vi "ADAM_info_to_Raw_data_header.vi"(4 "Results file":path) -> ()   [LabVIEW 2010]
panel:
  out "ADAM Channel Info":string[][](table)
  out "Raw data filenames":string[](array[string])
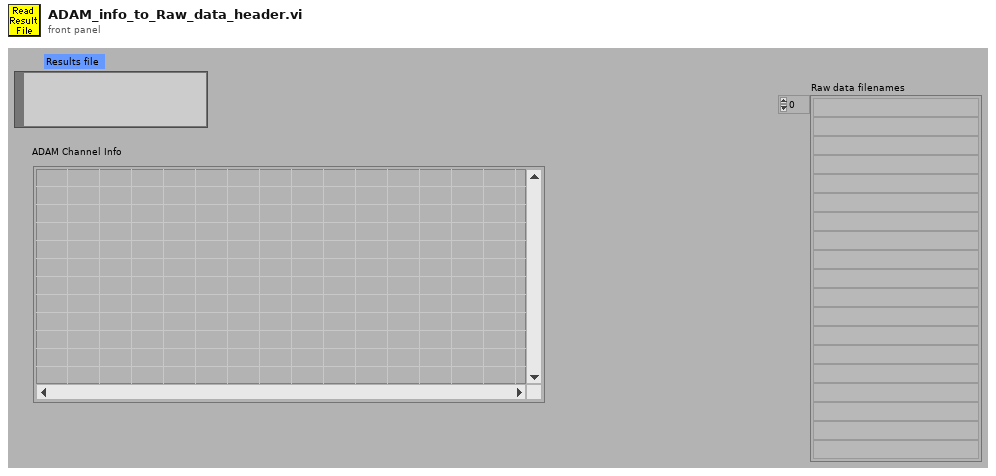
[diagram p1: front panel]
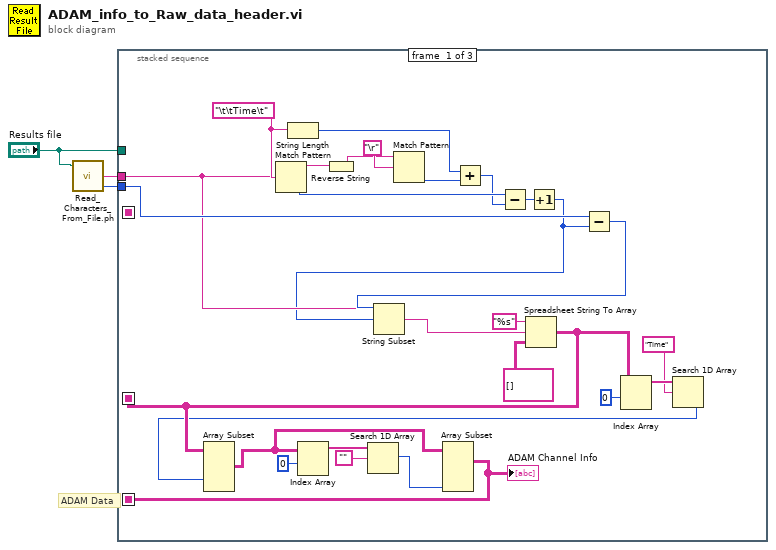
[diagram p0: block diagram]
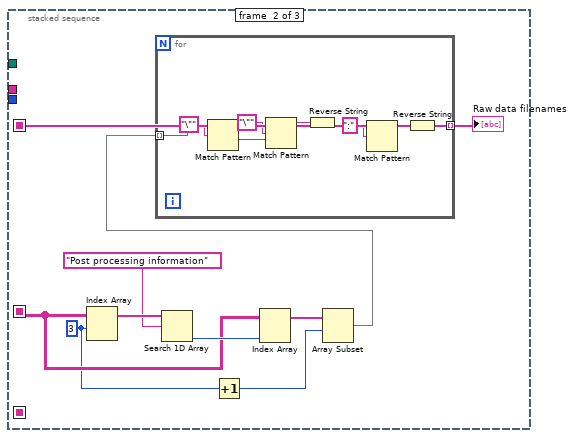
[diagram p2: hidden frame]
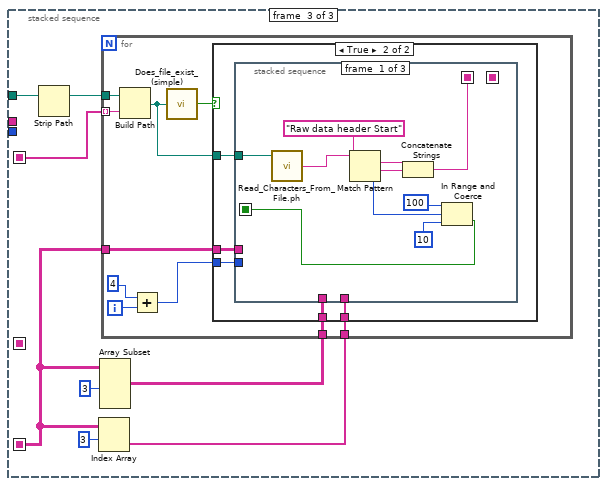
[diagram p3: hidden frame]
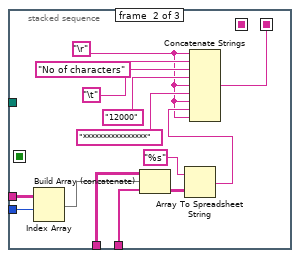
[diagram p5: hidden frame]
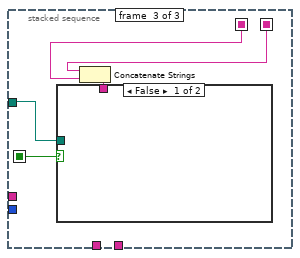
[diagram p6: hidden frame]
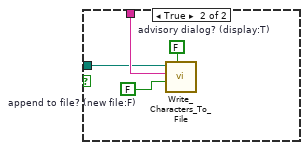
[diagram p7: hidden frame]
diagram:
  # "ADAM Data"
  n1 = call "Read_Characters_From_File.ph.vi"("file path (dialog if empty)"="Results file") -> ("character string"=w3:string, "mark after read (chars.)"=w2:i32)  [unwired: 5 in, 2 out]
  n2 = stacked-sequence {
    seq-local: [w7 _ _] -> [_ w36 _]
    seq-local: [w9 _ _] -> [_ _ w51]
    seq-local: [_ w31 _] -> [_ _ w53]
    tunnel: w3 -> [w19 _ _]
    tunnel: w2 -> [w22 _ _]
    tunnel: "Results file" -> [_ _ w54]
    frame #0 {
      w27 = "\t\tTime\t" ("regular expression")
      n3 = Match Pattern(string=w19, regular expression=w27) -> (before substring=w30:string, offset past match=w24:i32)  [unwired: 1 in, 2 out]
      n4 = String Length(string=w27) -> (length=w25:i32)
      n5 = Reverse String(1:w30) -> (0:w28:string)
      n6 = Match Pattern(string=w28, regular expression="\r") -> (offset past match=w26:i32)  [unwired: 1 in, 3 out]
      n7 = Add(x=w25, y=w26) -> (x+y=w23:i32)
      n8 = Subtract(x=w24, y=w23) -> (x-y=w21:i32)
      n9 = Increment(x=w21) -> (x+1=w18:i32)
      n10 = Subtract(x=w22, y=w18) -> (x-y=w20:i32)
      n11 = String Subset(string=w19, offset (0)=w18, length (rest)=w20) -> (substring=w17:string)
      n12 = Spreadsheet String To Array(format string="%s", spreadsheet string=w17, array type (2D Dbl)=string[][] [] ("Values")) -> (array=w7:string[][])  [unwired: 1 in]
      n13 = Index Array(array=w7, index (row)=0 ("Index")) -> (element=w6:string[])  [unwired: 1 in]
      n14 = Search 1D Array(1D array=w6, element="Time") -> (index of element=w4:i32)  [unwired: 1 in]
      n15 = Array Subset(array=w7, index (col)=w4) -> (w11:string[][])  [unwired: 3 in]
      n16 = Index Array(array=w11, index (row)=0 ("Index")) -> (element=w13:string[])  [unwired: 1 in]
      n17 = Search 1D Array(1D array=w13, element="") -> (index of element=w10:i32)  [unwired: 1 in]
      n18 = Array Subset(array=w11, length (col)=w10) -> (w9:string[][])  [unwired: 3 in]
      "ADAM Channel Info" <- w9
    }
    frame #1 {
      w35 = 3 ("Index")
      n19 = Index Array(array=w36, index (row)=w35) -> (element=w39:string[])  [unwired: 1 in]
      n20 = Search 1D Array(1D array=w39, element="Post processing information") -> (index of element=w37:i32)  [unwired: 1 in]
      n21 = Increment(x=w35) -> (x+1=w33:i32)
      n22 = Index Array(array=w36, index (col)=w37) -> (element=w34:string[])  [unwired: 1 in]
      n23 = Array Subset(array=w34, index=w33) -> (w32:string[])  [unwired: 1 in]
      n24 = for {
        tunnel: w32 -> [w47] mode=indexing
        tunnel: [w40] -> w31 mode=indexing
        n25 = Match Pattern(string=w47, regular expression="\"") -> (after substring=w45:string)  [unwired: 1 in, 3 out]
        n26 = Match Pattern(string=w45, regular expression="\"") -> (before substring=w44:string)  [unwired: 1 in, 3 out]
        n27 = Reverse String(1:w44) -> (0:w42:string)
        n28 = Match Pattern(string=w42, regular expression=":") -> (before substring=w41:string)  [unwired: 1 in, 3 out]
        n29 = Reverse String(1:w41) -> (0:w40:string)
      }
      "Raw data filenames" <- w31
    }
    frame #2 {
      n30 = Strip Path(path=w54) -> (stripped path=w52:path)  [unwired: 1 out]
      n31 = Index Array(array=w51, index (row)=3 ("Index")) -> (element=w49:string[])  [unwired: 1 in]
      n32 = Array Subset(array=w51, length (row)=3 ("Array Length")) -> (w50:string[][])  [unwired: 3 in]
      n33 = for {
        tunnel: w53 -> [w64] mode=indexing
        tunnel: w52 -> [w63]
        tunnel: w51 -> [w59]
        tunnel: w50 -> [w58]
        tunnel: w49 -> [w57]
        i -> [w66]
        n34 = Build Path(base path=w63, name or relative path=w64) -> (appended path=w61:path)
        n35 = Add(x=4 ("Index"), y=w66) -> (x+y=w60:i32)
        n36 = call "Does_file_exist_(simple).vi"("Pathname"=w61) -> ("exists?"=w62:bool)
        n37 = case shown="True" w62 {
          tunnel: w61 -> [_ w71]
          tunnel: w60 -> [_ w70]
          tunnel: w59 -> [_ w69]
          tunnel: w58 -> [_ w68]
          tunnel: w57 -> [_ w67]
          frame False {
          }
          frame True {
            n38 = stacked-sequence {
              seq-local: [w76 _ _] -> [_ _ w100]
              seq-local: [_ w84 _] -> [_ _ w99]
              seq-local: [w75 _ _] -> [_ _ w96]
              tunnel: w71 -> [w81 _ w97]
              tunnel: w70 -> [_ w95 _]
              tunnel: w69 -> [_ w94 _]
              tunnel: w68 -> [_ w93 _]
              tunnel: w67 -> [_ w92 _]
              frame #0 {
                n39 = call "Read_Characters_From_File.ph.vi"("file path (dialog if empty)"=w81) -> ("character string"=w79:string)  [unwired: 5 in, 3 out]
                n40 = Match Pattern(string=w79, regular expression="Raw data header Start") -> (match substring=w78:string, after substring=w77:string, offset past match=w74:i32)  [unwired: 1 in, 1 out]
                n41 = Concatenate Strings(w78, w77) -> (w76:string)
                n42 = In Range and Coerce(upper limit=100 ("y"), x=w74, lower limit=10 ("y")) -> (In Range?=w75:bool)  [unwired: 1 out]
              }
              frame #1 {
                w82 = "\r"
                n43 = Index Array(array=w94, index (row)=w95) -> (element=w91:string[])  [unwired: 1 in]
                n44 = Build Array (concatenate)(w93, w91, w92) -> (w90:string[][])
                n45 = Array To Spreadsheet String(array=w90, 3:"%s" ("format string")) -> (spreadsheet string=w83:string)  [unwired: 1 in]
                n46 = Concatenate Strings(w82, "No of characters", "\t", "12000" ("Substring"), w82, "****************" ("Substring"), w82, w83, w82) -> (w84:string)
              }
              frame #2 {
                n47 = Concatenate Strings(w99, w100) -> (w98:string)
                n48 = case shown="False" w96 {
                  tunnel: w98 -> [_ w104]
                  tunnel: w97 -> [_ w103]
                  frame False {
                  }
                  frame True {
                    w101 = FALSE  # append to file? (new file:F)
                    w102 = FALSE  # advisory dialog? (display:T)
                    n49 = call "Write_Characters_To_File.vi"("file path (dialog if empty)"=w103, "advisory dialog? (display:T)"=w102, "character string"=w104, "append to file? (new file:F)"=w101) -> ()  [unwired: 4 in, 1 out]
                  }
                }
              }
            }
          }
        }
      }
    }
  }
